vi "GOMDBTS2048 get Number Of Pixel.vi"(8 "error in (no error)":errorcluster) -> (0 "error out":errorcluster, 2 "function return":i32, 3 "nr of pixel":i32)   [LabVIEW 2015, in "GOMDBTS2048.lvlib"]
doc: "GOBTS2048DLL int __stdcall GOMDBTS2048_getHandle(char* device, int* handle);"
uses:
  GOMDBTS2048.lvlib
  runtime/GOMDBTS2048.dll
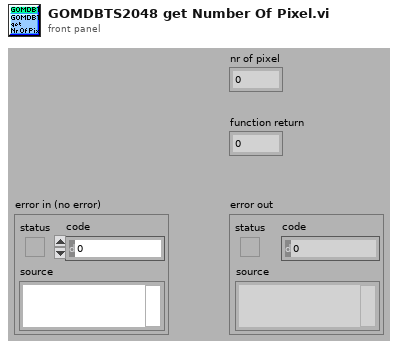
[diagram p1: front panel]
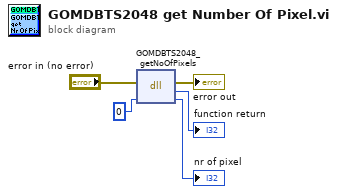
[diagram p0: block diagram]
diagram:
  n1 = dll-call lib="C:/Users/rkoch/Documents/GO_Library/runtime/GOMDBTS2048.*" fn="GOMDBTS2048_getNoOfPixels"(error in="error in (no error)", "nr of pixel"=0 ("handle")) -> (error out=→"error out":errorcluster, "return type"=→"function return":i32, "nr of pixel"=→"nr of pixel":i32)  [unwired: 2 in, 1 out]
